vi "FSM_sensor_switch.vi"(0 "Sensor 1":dbl, 1 "Sensor 2":dbl, 3 "h_min":dbl, 4 "h_max":dbl, 7 "error in (no error)":errorcluster, 10 "Sensor_inicial":u16(ring) items=["sensor_1", "sensor_2"], 11 "Period":i64=100, 15 "Priority":i32=3, 16 "stop":bool) -> (20 "y":dbl(graph), 22 "Sensor":u16, 27 "error out":errorcluster)   [LabVIEW 2019]
panel:
  in  "Tab Control":enum32{"Painel Frontal", "Diagramas"}(tab)
  # "Início"
  # "y > h_max"
  # "SENSOR 1"
  # "SENSOR 2"
  # "h_min<= y <= h_max"
  # "h_min<= y <= h_max"
  # "y < h_min"
  # "sensor 2"
  # "y > h_max"
  # "y < h_min"
  # "sensor 1"
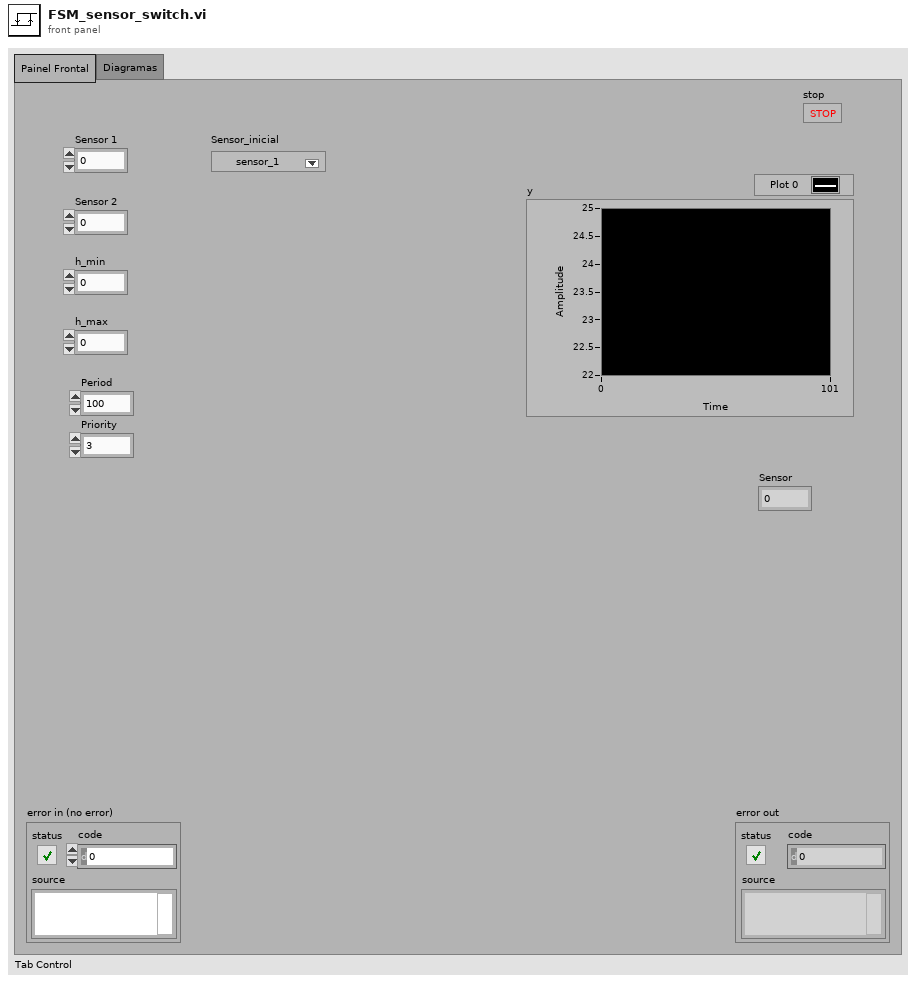
[diagram p1: front panel]
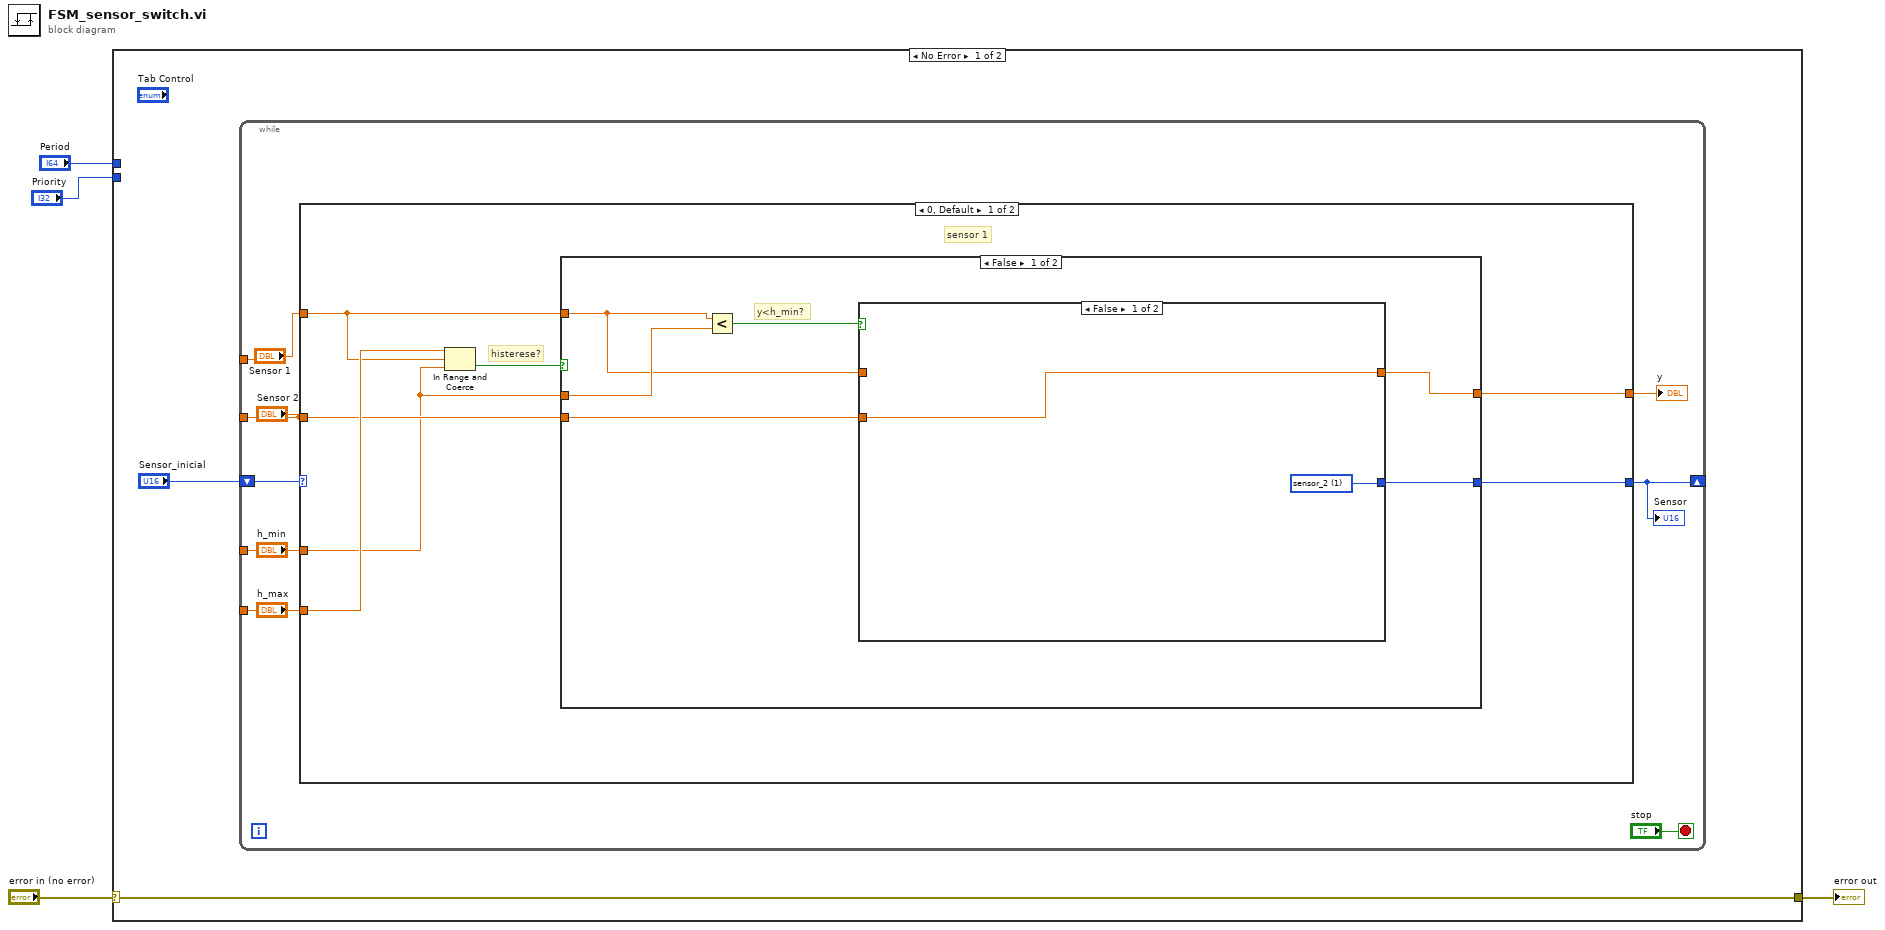
[diagram p0: block diagram]
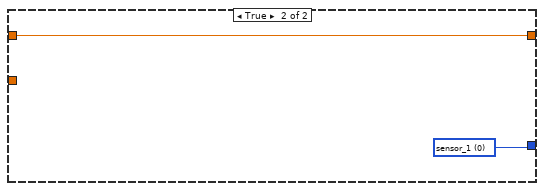
[diagram p2: hidden frame]
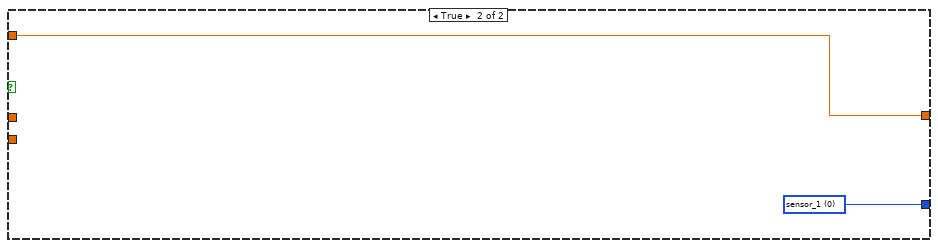
[diagram p3: hidden frame]
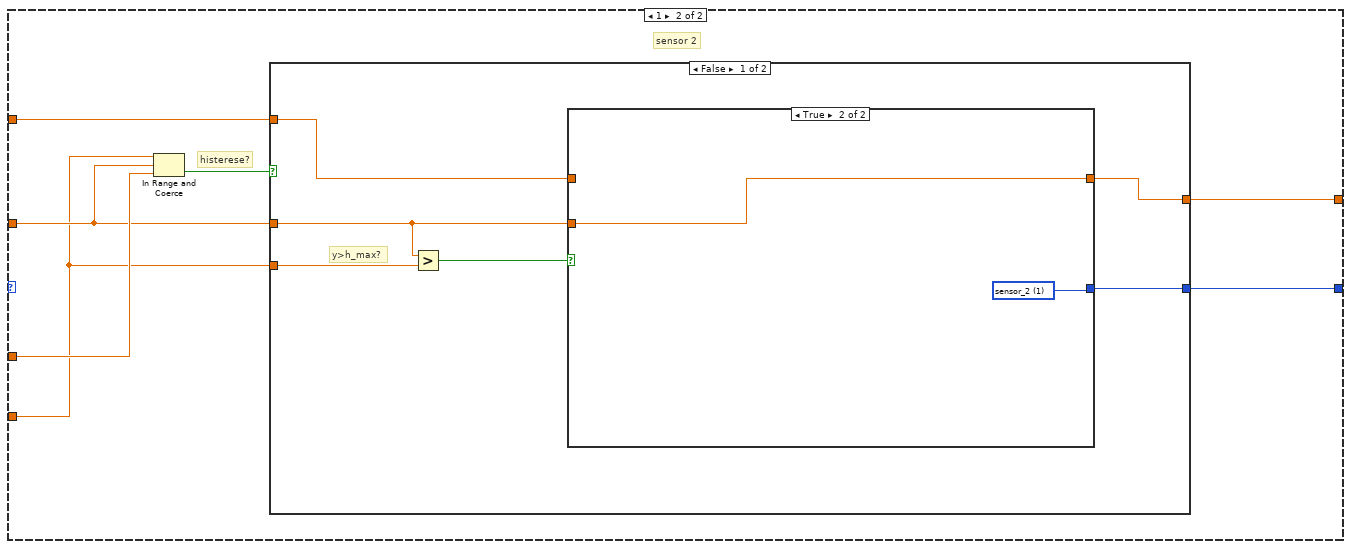
[diagram p4: hidden frame]
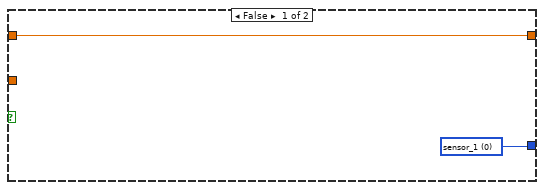
[diagram p5: hidden frame]
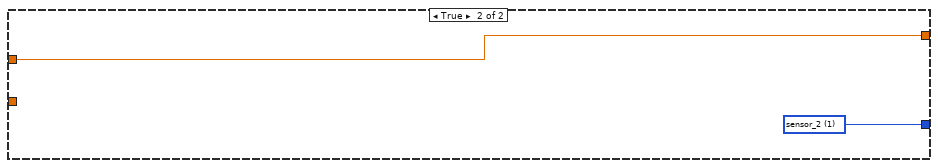
[diagram p6: hidden frame]
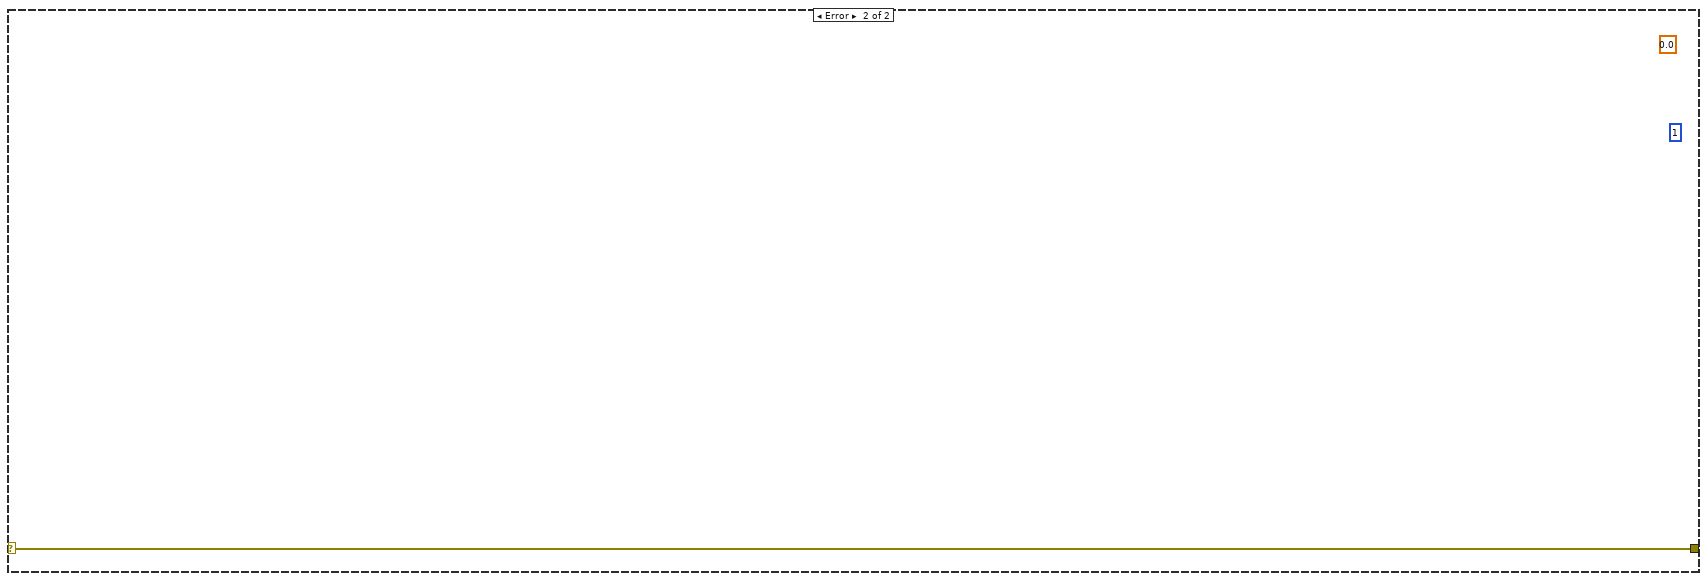
[diagram p7: hidden frame]
diagram:
  n1 = case shown="No Error" "error in (no error)" {
    selector: "error in (no error)" -> [w6 w53]
    tunnel: [w6 w53] -> w3
    tunnel: "Period" -> [_ _]
    tunnel: "Priority" -> [_ _]
    frame No Error {
      n2 = while {
        shift-right: [w7] -> _
        shift-left: "Sensor_inicial" -> [w14]
        tunnel: ["h_min"] -> _
        tunnel: ["h_max"] -> _
        tunnel: ["Sensor 1"] -> _
        tunnel: ["Sensor 2"] -> _
        stop <- "stop" stop-if-true
        n3 = case shown="0, Default" w14 {
          tunnel: "h_min" -> [w15 w36]
          tunnel: "h_max" -> [w21 w34]
          tunnel: "Sensor 1" -> [w18 w38]
          tunnel: "Sensor 2" -> [w17 w35]
          tunnel: [w19 w39] -> w7
          tunnel: [w16 w37] -> w12
          frame 0, Default {
            # "histerese?"
            # "sensor 1"
            n4 = In Range and Coerce(upper limit=w21, x=w18, lower limit=w15) -> (In Range?=w20:bool)  [unwired: 1 out]
            n5 = case shown="False" w20 {
              tunnel: [w22 w33] -> w19
              tunnel: w18 -> [w25 w32]
              tunnel: w17 -> [w24 _]
              tunnel: [w23 w32] -> w16
              tunnel: w15 -> [w27 _]
              frame False {
                # "y<h_min?"
                n6 = Less?(x=w25, y=w27) -> (x < y?=w26:bool)
                n7 = case shown="False" w26 {
                  tunnel: w25 -> [_ w31]
                  tunnel: w24 -> [w29 _]
                  tunnel: [w29 w31] -> w23
                  tunnel: [w28 w30] -> w22
                  frame False {
                    w28 = u16 1 items=["sensor_1", "sensor_2"] ("Sensor_inicial")
                  }
                  frame True {
                    w30 = u16 0 items=["sensor_1", "sensor_2"] ("Sensor_inicial")
                  }
                }
              }
              frame True {
                w33 = u16 0 items=["sensor_1", "sensor_2"] ("Sensor_inicial")
              }
            }
          }
          frame 1 {
            # "histerese?"
            # "sensor 2"
            n8 = In Range and Coerce(upper limit=w34, x=w35, lower limit=w36) -> (In Range?=w40:bool)  [unwired: 1 out]
            n9 = case shown="False" w40 {
              tunnel: [w42 w52] -> w39
              tunnel: w38 -> [w44 _]
              tunnel: w35 -> [w41 w51]
              tunnel: [w43 w51] -> w37
              tunnel: w34 -> [w46 _]
              frame False {
                # "y>h_max?"
                n10 = Greater?(x=w41, y=w46) -> (0:w45:bool)
                n11 = case shown="True" w45 {
                  tunnel: w44 -> [w47 _]
                  tunnel: w41 -> [_ w49]
                  tunnel: [w47 w49] -> w43
                  tunnel: [w48 w50] -> w42
                  frame False {
                    w48 = u16 0 items=["sensor_1", "sensor_2"] ("Sensor_inicial")
                  }
                  frame True {
                    w50 = u16 1 items=["sensor_1", "sensor_2"] ("Sensor_inicial")
                  }
                }
              }
              frame True {
                w52 = u16 1 items=["sensor_1", "sensor_2"] ("Sensor_inicial")
              }
            }
          }
        }
        "y" <- w12
        "Sensor" <- w7
      }
    }
    frame Error {
      (unwired) u16 1 ("Sensor_inicial")
      (unwired) 0.0 ("Sensor 2")
    }
  }
  "error out" <- w3
